vi "solar_misc xml Attribute.vi"(10 "Name":string, 11 "Attributes (Name, Value)":string[][](array[string])) -> (2 "Found?":bool, 3 "Value":string)   [LabVIEW 2018]
doc: "This VI returns an XML attributes value"
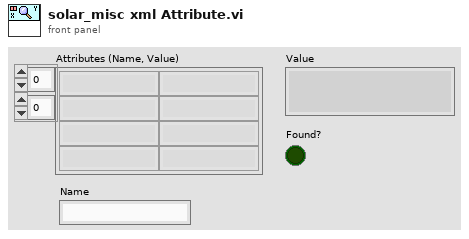
[diagram p1: front panel]
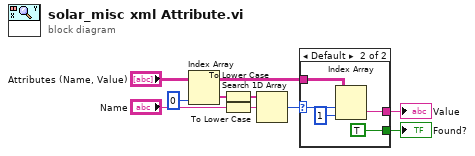
[diagram p0: block diagram]
diagram:
  n1 = Index Array(array="Attributes (Name, Value)", index (col)=0 ("disabled index (col)")) -> (element=w4:string[])  [unwired: 1 in]
  n2 = To Lower Case(string=w4) -> (all lower case string=w5:string[])
  n3 = To Lower Case(string="Name") -> (all lower case string=w8:string)
  n4 = Search 1D Array(1D array=w5, element=w8) -> (index of element=w2:i32)  [unwired: 1 in]
  n5 = case shown="Default" w2 {
    selector: w2 -> [_ w12]
    tunnel: [_ w10] -> w9
    tunnel: "Attributes (Name, Value)" -> [_ w13]
    tunnel: [_ TRUE] -> w1
    frame -1 {
    }
    frame Default {
      n6 = Index Array(array=w13, index (row)=w12, index (col)=1 ("disabled index (col)")) -> (element=w10:string)
    }
  }
  "Value" <- w9
  "Found?" <- w1
